vi "数据库路径确认.vi"(10 "选项":enum16{"初始化", "读取"}(ring)) -> (2 "数据库路径":path)   [LabVIEW 2017]
uses:
  Sqlite/CBB/CreatTable.vi
  Sqlite/SQLite.lvlib
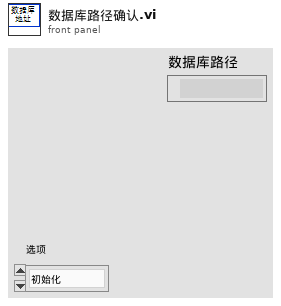
[diagram p1: front panel]
types:
  T1 = cluster{"设备明细":cluster{"table":string, "column":string[]}, "ER":cluster{"table":string, "column":string[]}}
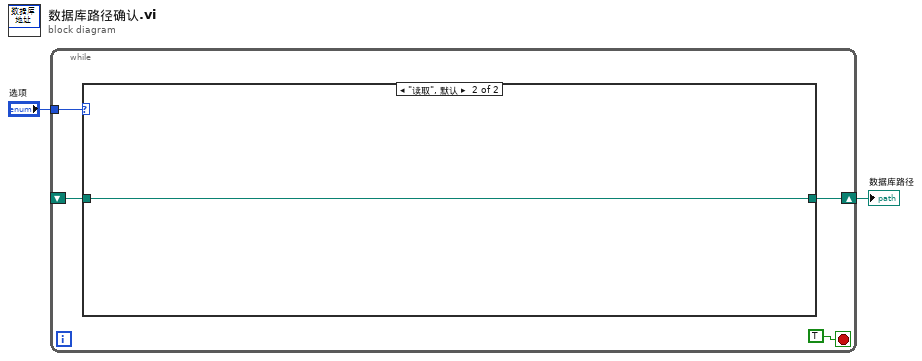
[diagram p0: block diagram]
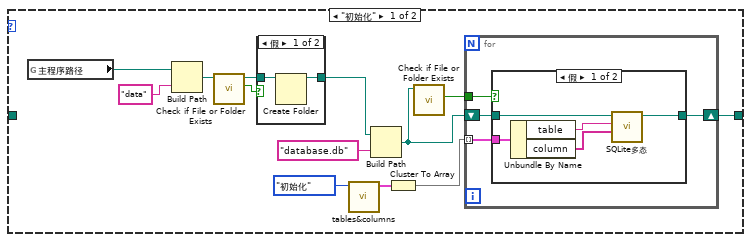
[diagram p2: hidden frame]
diagram:
  n1 = while {
    shift-right: [w5] -> w1
    shift-left: _ -> [w4]
    tunnel: "选项" -> [w3]
    stop <- TRUE stop-if-true
    n2 = case shown="\"读取\", 默认" w3 {
      tunnel: [w9 w33] -> w5
      tunnel: w4 -> [_ w33]
      frame "初始化" {
        n3 = global read "全局 1.vi" "主程序路径"() -> (w8:path)
        n4 = Build Path(base path=w8, name or relative path="data" ("名称或相对路径")) -> (appended path=w15:path)
        n5 = call <vilib>:"Check if File or Folder Exists.vi"("path"=w15) -> ("file or folder exists?"=w14:bool, "dup path"=w13:path)  [unwired: 8 in, 1 out]
        n6 = case shown="假" w14 {
          tunnel: [w30 w32] -> w12
          tunnel: w13 -> [w31 w32]
          frame False {
            n7 = Create Folder(path (use dialog)=w31) -> (created path=w30:path)  [unwired: 2 in, 2 out]
          }
          frame True {
          }
        }
        n8 = call "tables&columns.vi"("选项"=enum16{"初始化", "获取寄存器"}."初始化") -> ("Tables&columns"=w10:T1)  [unwired: 9 in, 1 out]
        n9 = Build Path(base path=w12, name or relative path="database.db" ("名称或相对路径")) -> (appended path=w17:path)
        n10 = Cluster To Array(cluster=w10) -> (array=w7:cluster{"table":string, "column":string[]}[])
        n11 = call <vilib>:"Check if File or Folder Exists.vi"("path"=w17) -> ("file or folder exists?"=w18:bool)  [unwired: 8 in, 2 out]
        n12 = for {
          tunnel: w18 -> [w23]
          tunnel: w7 -> [w21] mode=indexing
          shift-right: [w20] -> w9
          shift-left: w17 -> [w22]
          n13 = case shown="假" w23 {
            tunnel: w22 -> [w28 w29]
            tunnel: [w27 w29] -> w20
            tunnel: w21 -> [w26 _]
            frame False {
              n14 = Unbundle By Name(w26) -> ("table"=w25:string, "column"=w24:string[])
              n15 = call-poly "SQLite多态.vi"("Columns"=w24, "Table Name"=w25, "DbPath"=w28) -> ("DbPath out"=w27:path)  [unwired: 6 in, 2 out]
            }
            frame True {
            }
          }
        }
      }
      frame "读取", Default {
      }
    }
  }
  "数据库路径" <- w1
